vi "custom_command_test.vi"() -> ()   [LabVIEW 2017]
uses:
  <vilib>/MakerHub/LINX/Public/Peripherals/Digital/Digital Read 1 Chan.vi
  <extravilib>/ChannelInstances/Stream-bool/Read With Abort.vi
  <extravilib>/ChannelInstances/Stream-bool/Write With Abort.vi
  <vilib>/MakerHub/LINX/Public/Peripherals/Digital/Digital Read N Chans.vi
  <extravilib>/ChannelInstances/Stream-bool/EndpointRead.vi
  <extravilib>/ChannelInstances/Stream-bool/Endpoint.vi
  <vilib>/MakerHub/LINX/Private/Local IO/LinxDigitalRead.vi
  <vilib>/MakerHub/LINX/Public/Utilities/Check Channel.vi
  <vilib>/MakerHub/LINX/Public/Utilities/Open Serial.vi
  <extravilib>/ChannelInstances/Stream-bool/Instantiate.vi
  <extravilib>/ChannelInstances/Stream-bool/)Channel.vi
  <resource>/ChannelSupport/_ChannelSupport/WaitIfNeeded.vi
  <vilib>/MakerHub/LINX/Private/Utilties/Generate Error.vi
  <vilib>/MakerHub/LINX/LMH-LINX.lvlib
  <extravilib>/ChannelInstances/Stream-bool.lvlib
panel:
  in  "Line 1":string
  in  "Line 0":string
  out "step size":dbl
  out "DI Value":bool
  out "step down":bool[](array[boolean])
  out "step up":bool[](array[boolean])
  in  "stop":bool
  out "Response":u8[](array[numeric])
  in  "Data":u8[](array[numeric])
  in  "Timeout (100 ms)":i32=100
  in  "Serial Port":refnum<visa-resource-name>="N/A"
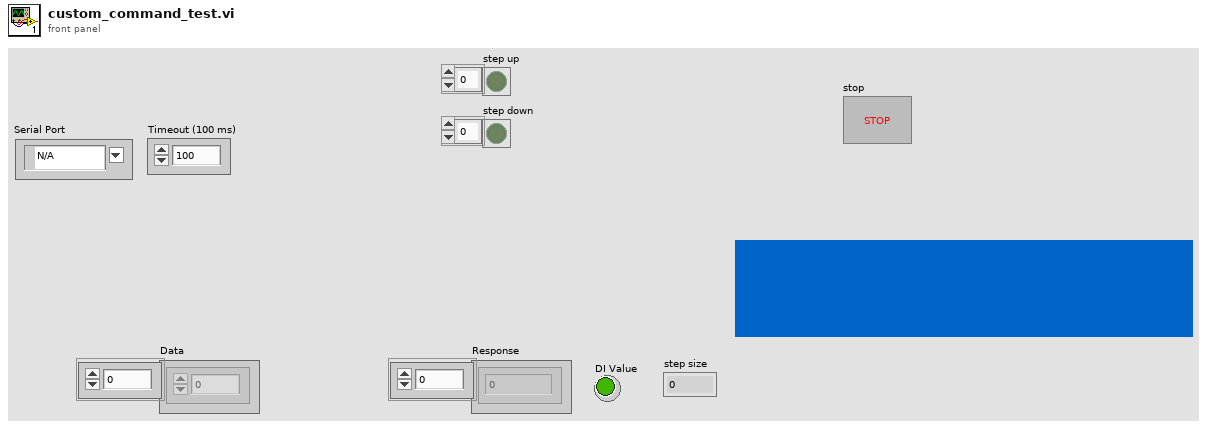
[diagram p1: front panel]
types:
  T1 = typedef "LMH-LINX.lvlib/LINX Ref.ctl" = cluster{"IO":T2, "Interface":T3, "LINX Device Config":T4}
  T2 = typedef "LMH-LINX.lvlib/Platform.ctl" = enum16{"Remote", "Local"}
  T3 = typedef "LMH-LINX.lvlib/Interface.ctl" = enum16{"Serial", "TCP"}
  T4 = typedef "LMH-LINX.lvlib/Device.lvlib/LINX Device Config.ctl" = cluster{"Interface":T3, "COM Port":refnum<visa-resource-name>, "TCP Configuration":T5, "Device Family":u8, "Device ID":u8, "Device Name":string, "TCP Ref":refnum<k5>, "Channels":T6}
  T5 = typedef "LMH-LINX.lvlib/Device.lvlib/TCP Config.ctl" = cluster{"IP Address":string, "Port":u16}
  T6 = typedef "LMH-LINX.lvlib/Channels.ctl" = cluster{"DI":u8[], "DO":u8[], "AI":u8[], "AO":u8[], "PWM":u8[], "QE":u8[], "UART":u8[], "I2C 2":u8[], "SPI":u8[], "CAN":u8[], "Servo":u8[], "AI Ref (V)":dbl, "AI Resolution (Bits)":u8, "AO Ref (V)":dbl, "AO Resolution (Bits)":u8}
  T7 = typedef "Stream-bool.lvlib/)Channel.ctl" = refnum<queue>
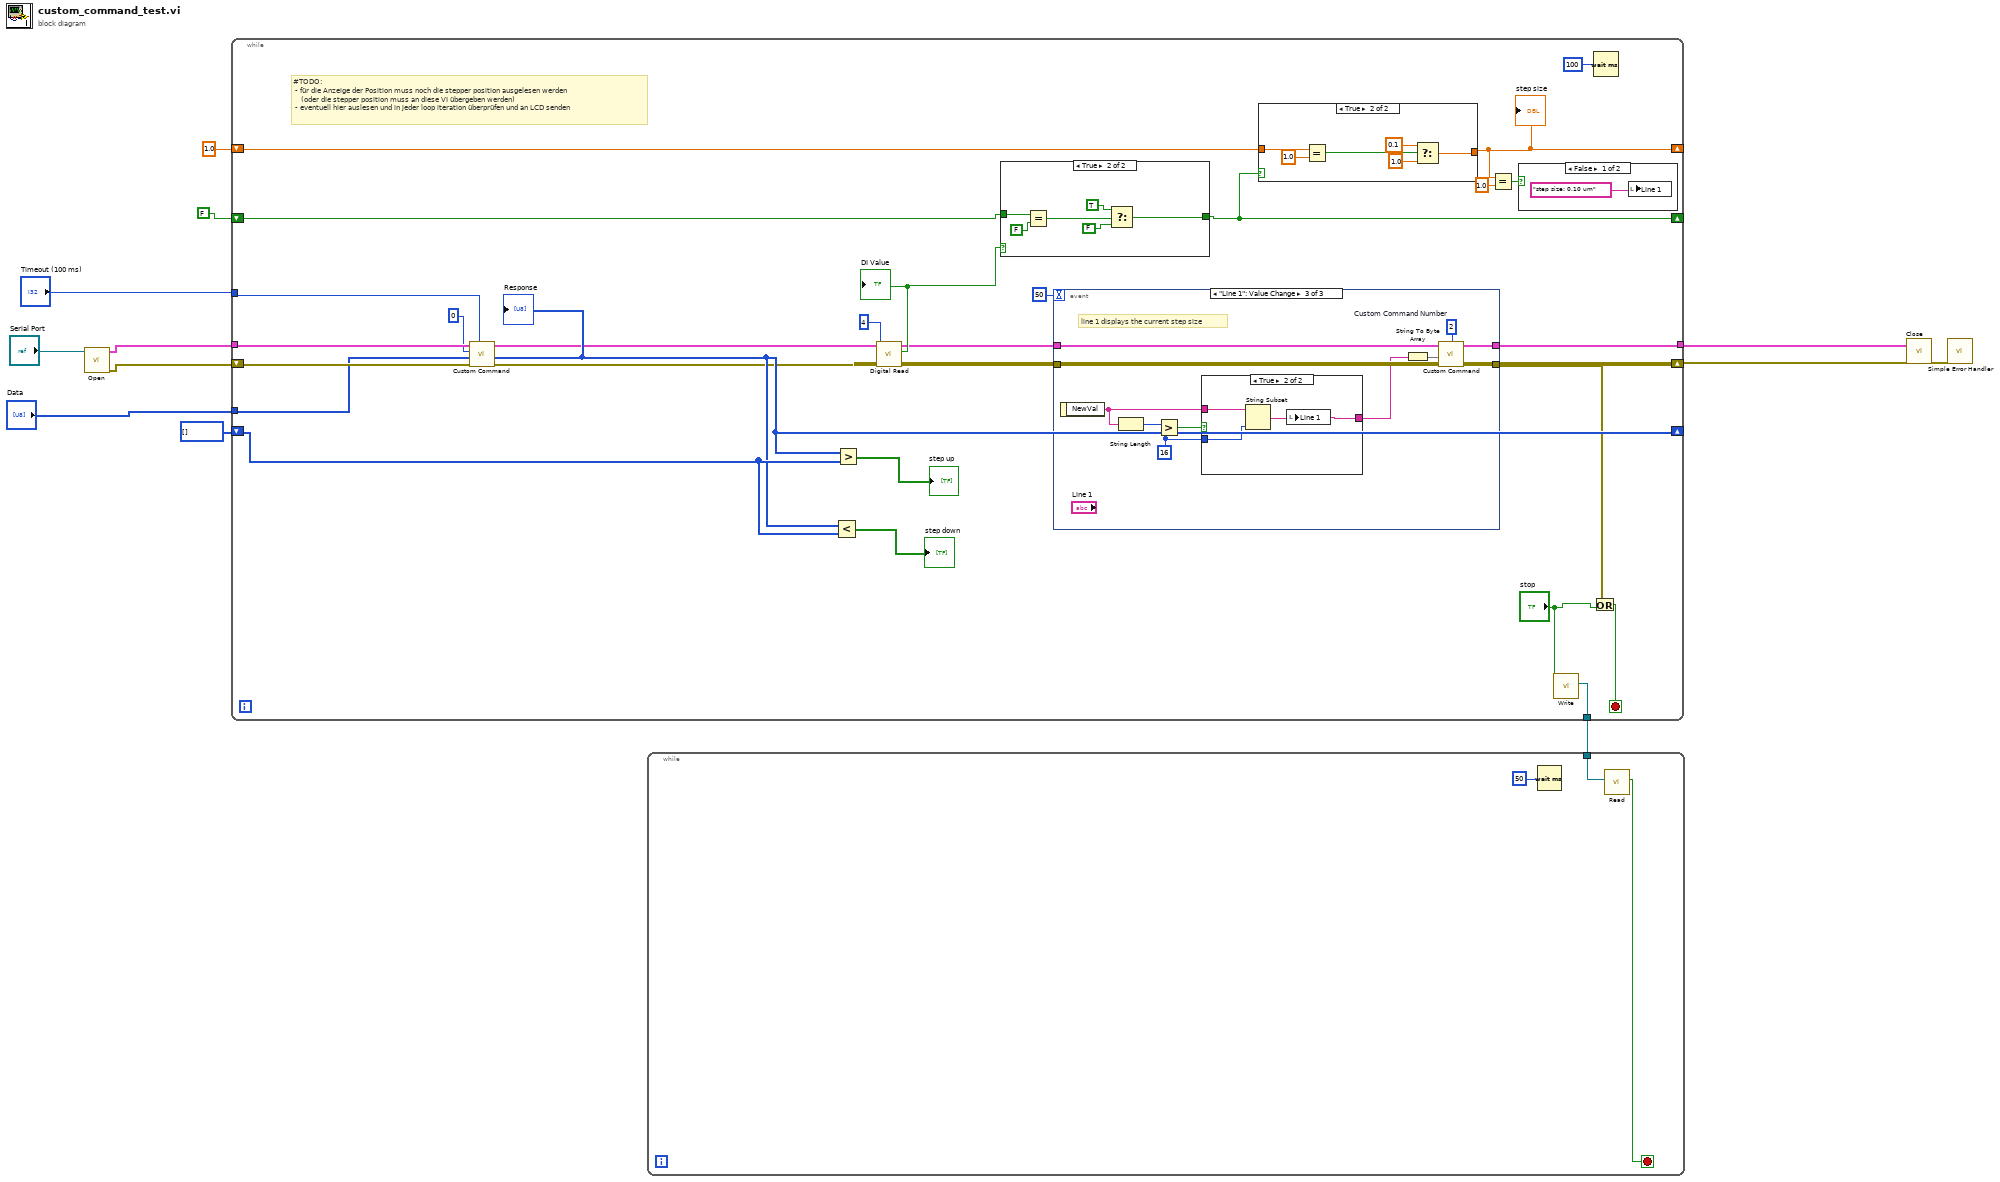
[diagram p0: block diagram]
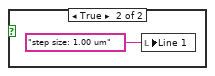
[diagram p2: hidden frame]
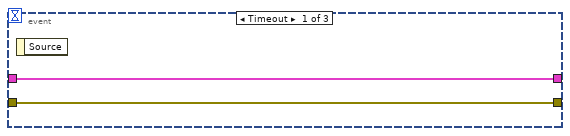
[diagram p3: hidden frame]
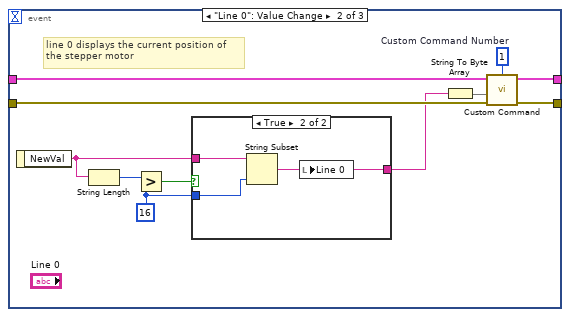
[diagram p4: hidden frame]
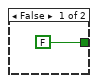
[diagram p7: hidden frame]
diagram:
  n1 = call-poly <vilib>:"Open.vi"("Serial Port"="Serial Port") -> ("Error Out"=w11:errorcluster, "LINX Resource"=w10:T1)  [unwired: 8 in, 1 out]
  n2 = while {
    tunnel: "Timeout (100 ms)" -> [w37]
    shift-right: [w17] -> w9
    shift-left: w11 -> [w39]
    tunnel: "Data" -> [w36]
    shift-right: [w32] -> _
    shift-left: u8[] [] ("Response") -> [w33]
    tunnel: w10 -> [w38]
    tunnel: [w18] -> w8
    tunnel: [w25] -> w3
    shift-right: [w14] -> _
    shift-left: 1.0 -> [w24]
    shift-right: [w21] -> _
    shift-left: FALSE -> [w22]
    stop <- w27 stop-if-true
    # "#TODO:\n - für die Anzeige der Position muss noch die stepper position ausgelesen werden\n    (oder die stepper position muss an diese VI übergeben werden)\n - eventuell hier auslesen und in jeder loop iteration überprüfen und an LCD senden"
    n3 = call <vilib>:"Custom Command.vi"("Timeout (100 ms)"=w37, "Error In"=w39, "Data"=w36, "Custom Command Number"=u16 0, "LINX Resource"=w38) -> ("Error Out"=w29:errorcluster, "Response"=w32:u8[], "LINX Resource"=w30:T1)  [unwired: 3 in, 1 out]
    "Response" <- w32
    n4 = Less?(x=w32, y=w33) -> (x < y?=→"step down":bool[])
    n5 = Greater?(x=w32, y=w33) -> (0:→"step up":bool[])
    n6 = call-poly <vilib>:"Digital Read.vi"("Error In"=w29, "DI Channel"=u8 4, "LINX Resource"=w30) -> ("Error Out"=w19:errorcluster, "DI Value"=w23:bool, "LINX Resource"=w20:T1)  [unwired: 6 in]
    "DI Value" <- w23
    n7 = case shown="True" w23 {
      tunnel: w22 -> [_ w81]
      tunnel: [FALSE w78] -> w21
      frame False {
      }
      frame True {
        n8 = Equal?(x=w81, y=FALSE) -> (x = y?=w80:bool)
        n9 = Select(t=TRUE, s=w80, f=FALSE) -> (s? t:f=w78:bool)
      }
    }
    n10 = event shown="[2] \"Line 1\": Value Change" {
      selector: _ -> [_ _ _]
      dyn-events: _ -> [_ _ _]
      timeout: 50 -> [_ _ _]
      tunnel: w20 -> [w44 w51 w66]
      tunnel: [w44 w49 w64] -> w18
      tunnel: [w43 w48 w63] -> w17
      tunnel: w19 -> [w43 w50 w65]
      event Timeout {
        n11 = event-data() -> ()  [unwired: 1 in, 1 out]
      }
      event "Line 0": Value Change {
        w45 = u16 1  # Custom Command Number
        w52 = 16 ("y")
        # "line 0 displays the current position of \nthe stepper motor"
        n12 = event-data() -> ("NewVal"=w53:string)  [unwired: 1 in]
        n13 = String Length(string=w53) -> (length=w55:i32)
        n14 = Greater?(x=w55, y=w52) -> (0:w54:bool)
        n15 = case shown="True" w54 {
          tunnel: w53 -> [w56 w59]
          tunnel: w52 -> [_ w58]
          tunnel: [w56 w57] -> w46
          frame False {
          }
          frame True {
            n16 = String Subset(string=w59, length (rest)=w58) -> (substring=w57:string)  [unwired: 1 in]
            n17 = local write "Line 0"(w57) -> ()
          }
        }
        n18 = String To Byte Array(string=w46) -> (unsigned byte array=w47:u8[])
        n19 = call <vilib>:"Custom Command.vi"("Error In"=w50, "Data"=w47, "Custom Command Number"=w45, "LINX Resource"=w51) -> ("Error Out"=w48:errorcluster, "LINX Resource"=w49:T1)  [unwired: 4 in, 2 out]
      }
      event "Line 1": Value Change {
        w60 = u16 2  # Custom Command Number
        w67 = 16 ("y")
        # "line 1 displays the current step size"
        n20 = event-data() -> ("NewVal"=w68:string)  [unwired: 1 in]
        n21 = String Length(string=w68) -> (length=w70:i32)
        n22 = Greater?(x=w70, y=w67) -> (0:w69:bool)
        n23 = case shown="True" w69 {
          tunnel: w68 -> [w71 w74]
          tunnel: w67 -> [_ w73]
          tunnel: [w71 w72] -> w61
          frame False {
          }
          frame True {
            n24 = String Subset(string=w74, length (rest)=w73) -> (substring=w72:string)  [unwired: 1 in]
            n25 = local write "Line 1"(w72) -> ()
          }
        }
        n26 = String To Byte Array(string=w61) -> (unsigned byte array=w62:u8[])
        n27 = call <vilib>:"Custom Command.vi"("Error In"=w65, "Data"=w62, "Custom Command Number"=w60, "LINX Resource"=w66) -> ("Error Out"=w63:errorcluster, "LINX Resource"=w64:T1)  [unwired: 4 in, 2 out]
      }
    }
    n28 = case shown="True" w21 {
      tunnel: [w82 w88] -> w14
      tunnel: w24 -> [w82 w87]
      frame False {
      }
      frame True {
        n29 = Equal?(x=w87, y=1.0) -> (x = y?=w85:bool)
        n30 = Select(t=0.1, s=w85, f=1.0) -> (s? t:f=w88:dbl)
      }
    }
    "step size" <- w14
    n31 = Equal?(x=w14, y=1.0) -> (x = y?=w15:bool)
    n32 = case shown="False" w15 {
      frame False {
        n33 = local write "Line 1"("step size: 0.10 um") -> ()
      }
      frame True {
        n34 = local write "Line 1"("step size: 1.00 um") -> ()
      }
    }
    n35 = call <extravilib>:"Write.vi"("element"="stop") -> ("channel"=w25:T7)  [unwired: 8 in, 2 out]
    n36 = Or(x=w17, y="stop") -> (x .or. y?=w27:bool)
    n37 = Wait (ms)(milliseconds to wait=u32 100) -> ()  [unwired: 1 out]
  }
  n38 = while {
    tunnel: w3 -> [w91]
    stop <- w90 stop-if-true
    n39 = Wait (ms)(milliseconds to wait=u32 50) -> ()  [unwired: 1 out]
    n40 = call <extravilib>:"Read.vi"("channel"=w91) -> ("element"=w90:bool)  [unwired: 6 in, 4 out]
  }
  n41 = call <vilib>:"Close.vi"("Error In"=w9, "LINX Resource"=w8) -> ("Error Out"=w4:errorcluster)  [unwired: 9 in]
  n42 = call <vilib>:"Simple Error Handler.vi"("error in (no error)"=w4) -> ()  [unwired: 4 in, 5 out]
